vi "Velocity Lifter PID.vi"(8 "MechanismMetrics":T1={"lift height"=0.0, "Command"=enum."Noop", "Time Stamp"=0, "ToggleCollector"=FALSE, "Bottom_Limit_Switch "=FALSE, "Top_Limit_Switch"=FALSE, "lift power"=0.0, "Elevator soleniod debounce time   "=3038815.0, "LifterOverride"=TRUE, "Previous Lift power"=0.0, "manual lift"=0.0, "Lifter State"=enum."LifterClosed", "Auto Lifter State"=enum."Not Pressed", "Toggle Auto Lifter"=FALSE, "Wait Timer"=0.0, "HP Auto Indexer"=FALSE, "HP Auto Lifter State"=enum."Not Pressed", "Commanded Velocity"=0.0}) -> (0 "MechanismMetrics 2":T1={"lift height"=0.0, "Command"=enum."Noop", "Time Stamp"=0, "ToggleCollector"=FALSE, "Bottom_Limit_Switch "=FALSE, "Top_Limit_Switch"=FALSE, "lift power"=0.0, "Elevator soleniod debounce time   "=3038815.0, "LifterOverride"=TRUE, "Previous Lift power"=0.0, "manual lift"=0.0, "Lifter State"=enum."LifterClosed", "Auto Lifter State"=enum."Not Pressed", "Toggle Auto Lifter"=FALSE, "Wait Timer"=0.0, "HP Auto Indexer"=FALSE, "HP Auto Lifter State"=enum."Not Pressed", "Commanded Velocity"=0.0})   [LabVIEW 2014]
uses:
  MechanismMetrics.ctl
  Lifter States.ctl
  Auto Lifter States.ctl
  encoderData.vi
  limitSwitchGlobals.vi
  <vilib>/addons/control/pid/pid.llb/PID (DBL).vi
  <vilib>/addons/control/pid/NI_PID_pid.lvlib
panel:
  in  "derivative time (Td, min)":dbl
  in  "integral time (Ti, min)":dbl=0.0025
  in  "proportional gain (Kc)":dbl=0.00015
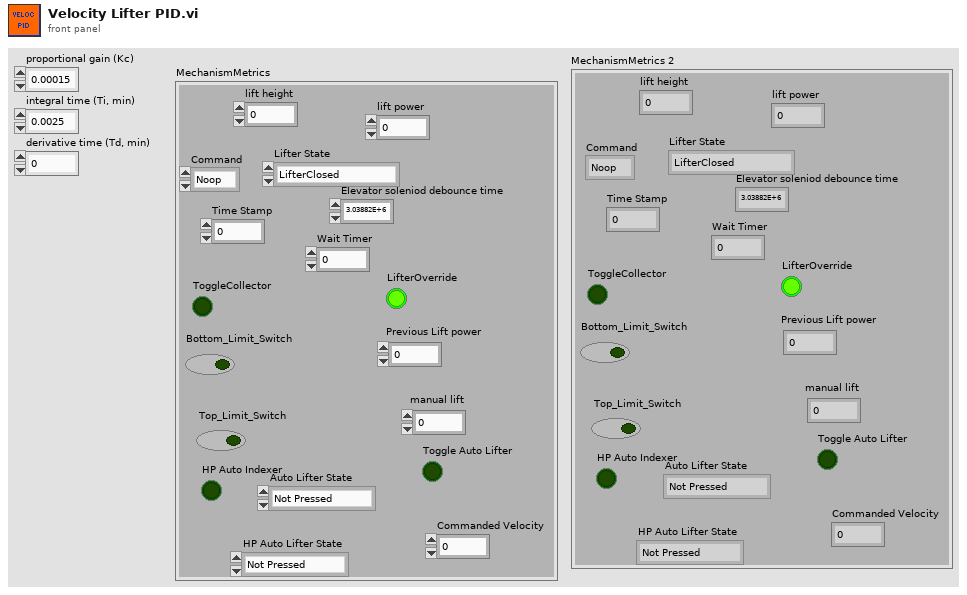
[diagram p1: front panel]
types:
  T1 = typedef "MechanismMetrics.ctl" = cluster{"lift height":dbl, "Command":enum16{"Noop", "Flagged"}, "Time Stamp":u32, "ToggleCollector":bool, "Bottom_Limit_Switch ":bool, "Top_Limit_Switch":bool, "lift power":dbl, "Elevator soleniod debounce time   ":dbl, "LifterOverride":bool, "Previous Lift power":dbl, "manual lift":dbl, "Lifter State":T2, "Auto Lifter State":T3, "Toggle Auto Lifter":bool, "Wait Timer":dbl, "HP Auto Indexer":bool, "HP Auto Lifter State":T3, "Commanded Velocity":dbl}
  T2 = typedef "Lifter States.ctl" = enum16{"OpeningLifter", "LifterOpen", "ClosingLifter", "LifterClosed"}
  T3 = typedef "Auto Lifter States.ctl" = enum16{"Not Pressed", "THE_END", "WAIT_FOR_RELEASE", "Press Detected", "To Release Stacked1", "To Collect", "Open Lifter", "WAIT", "Close", "To Stack1"}
  T4 = cluster{"proportional gain (Kc)":dbl, "integral time (Ti, min)":dbl, "derivative time (Td, min)":dbl}
  T5 = typedef "WPI_MotorControlDeviceRef.ctl" = cluster{"DeviceStatus":errorcluster, "Type":T6, "PWM":cluster{"Controller":T7, "PWM Channel":T8, "DeadBand":T9}, "CAN":cluster{"Device Number":u8, "Control Mode":T10, "Semaphore":T11, "Max Vout":dbl, "TalonSRX Control Mode":T12}, "Invert":bool, "TransformRef":T13, "InvTransformRef":T13}
  T6 = typedef "WPI_MotorControlType.ctl" = enum16{"PWM", "CAN", "CANTalonSRX"}
  T7 = typedef "FPGA_TypedefDigitalModule.ctl" = enum16{"Controller 1"}
  T8 = typedef "FPGA_DIOPWMChannel.ctl" = enum8{"PWM 0", "PWM 1", "PWM 2", "PWM 3", "PWM 4", "PWM 5", "PWM 6", "PWM 7", "PWM 8", "PWM 9", "PWM MXP 0", "PWM MXP 1", "PWM MXP 2", "PWM MXP 3", "PWM MXP 4", "PWM MXP 5", "PWM MXP 6", "PWM MXP 7", "PWM MXP 8", "PWM MXP 9", "Invalid"}
  T9 = typedef "WPI_PWMDeadband.ctl" = cluster{"Name":string, "maxPositivePwm":i32, "minPositivePwm":i32, "centerPwm":i32, "maxNegativePwm":i32, "minNegativePwm":i32, "angularRange":u16}
  T10 = typedef "WPI_CANJaguar_ControlMode.ctl" = enum8{"Percent VBus", "Current", "Speed", "Position", "Voltage"}
  T11 = typedef "Semaphore RefNum" = refnum<k1>
  T12 = typedef "WPI_CANTalonSRX_APIControlMode.ctl" = enum8{"Percent VBus", "Speed", "Position", "Slave", "Unchanged / Invalid"}
  T13 = typedef "WPI_PWMTransform_ConPane.ctl" = refnum<vi>
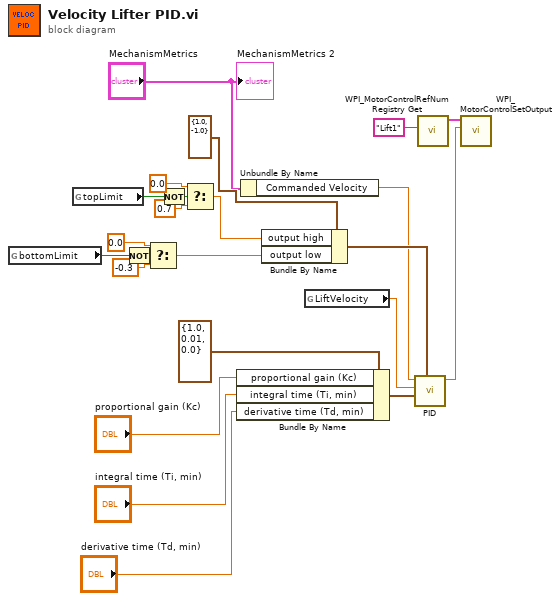
[diagram p0: block diagram]
diagram:
  n1 = global read "limitSwitchGlobals.vi" "bottomLimit"() -> (w3:bool)
  n2 = global read "limitSwitchGlobals.vi" "topLimit"() -> (w4:bool)
  n3 = Not(x=w3) -> (.not. x?=w1:bool)
  n4 = Select(t=0.0, s=w1, f=-0.3 ("output low")) -> (s? t:f=w16:dbl)
  n5 = Not(x=w4) -> (.not. x?=w2:bool)
  n6 = Select(t=0.0, s=w2, f=0.7 ("output high")) -> (s? t:f=w13:dbl)
  n7 = Bundle By Name(cluster=T4 {"proportional gain (Kc)"=1.0, "integral time (Ti, min)"=0.01, "derivative time (Td, min)"=0.0} ("PID gains"), "proportional gain (Kc)"="proportional gain (Kc)", "integral time (Ti, min)"="integral time (Ti, min)", "derivative time (Td, min)"="derivative time (Td, min)") -> (w22:T4)
  n8 = Unbundle By Name("MechanismMetrics") -> ("Commanded Velocity"=w18:dbl)
  n9 = Bundle By Name(cluster=cluster{"output high":dbl, "output low":dbl} {"output high"=1.0, "output low"=-1.0} ("output range"), "output high"=w13, "output low"=w16) -> (w20:cluster{"output high":dbl, "output low":dbl})
  n10 = global read "encoderData.vi" "LiftVelocity"() -> (w17:dbl)
  n11 = call-poly <vilib>:"PID.vi"("output range"=w20, "PID gains"=w22, "process variable"=w17, "setpoint"=w18) -> ("output"=w8:dbl)  [unwired: 6 in, 1 out]
  n12 = call <vilib>:"WPI_MotorControlRefNum Registry Get.vi"("refnum name"="Lift1") -> ("MotorControlDevRef"=w10:T5)  [unwired: 9 in, 1 out]
  n13 = call <vilib>:"WPI_MotorControlSetOutput.vi"("Output"=w8, "MotorControlDevRef"=w10) -> ()  [unwired: 7 in, 3 out]
  "MechanismMetrics 2" <- "MechanismMetrics"
